vi "pumpsec_09_P2.vi"(0 "reset":i32, 1 "master":i32, 4 "manual":i32, 5 "pause":i32, 10 "Array":dbl[](array[numeric]), 14 "Target":dbl[](array[numeric])=[10.0, 2.0, 0.0, 0.0, 0.0, 0.0, 0.0, 0.0, 0.0, 0.0], 16 "fr_manual":dbl, 17 "Time":dbl[](array[numeric])=[4.0, 2.0, 0.0, 0.0, 0.0, 0.0, 0.0, 0.0, 0.0, 0.0]) -> (2 "pumpCtrl":dbl, 3 "totaltarget":dbl, 6 "target_step":dbl, 7 "REGLO D":dbl, 11 "time_to_target":dbl, 12 "step_fr":dbl, 13 "amount_step":dbl, 19 "reset_out":dbl, 20 "Scale":dbl, 23 "elapsed_step":dbl, 24 "Scale actual":dbl, 25 "params":dbl[](array[numeric]))   [LabVIEW 2016]
uses:
  Desktop/Bertta-Bertta_deploy/Bertta-Bertta_deploy/BERTTA/x64/Debug/BERTTA.dll
panel:
  out "amount_step_previous":dbl
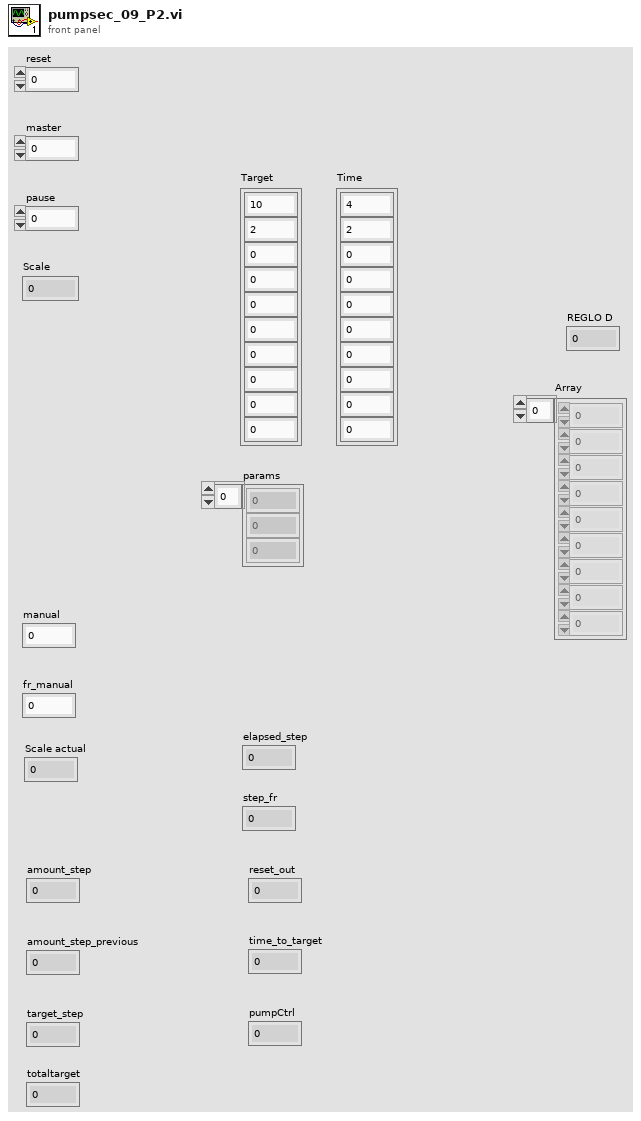
[diagram p1: front panel]
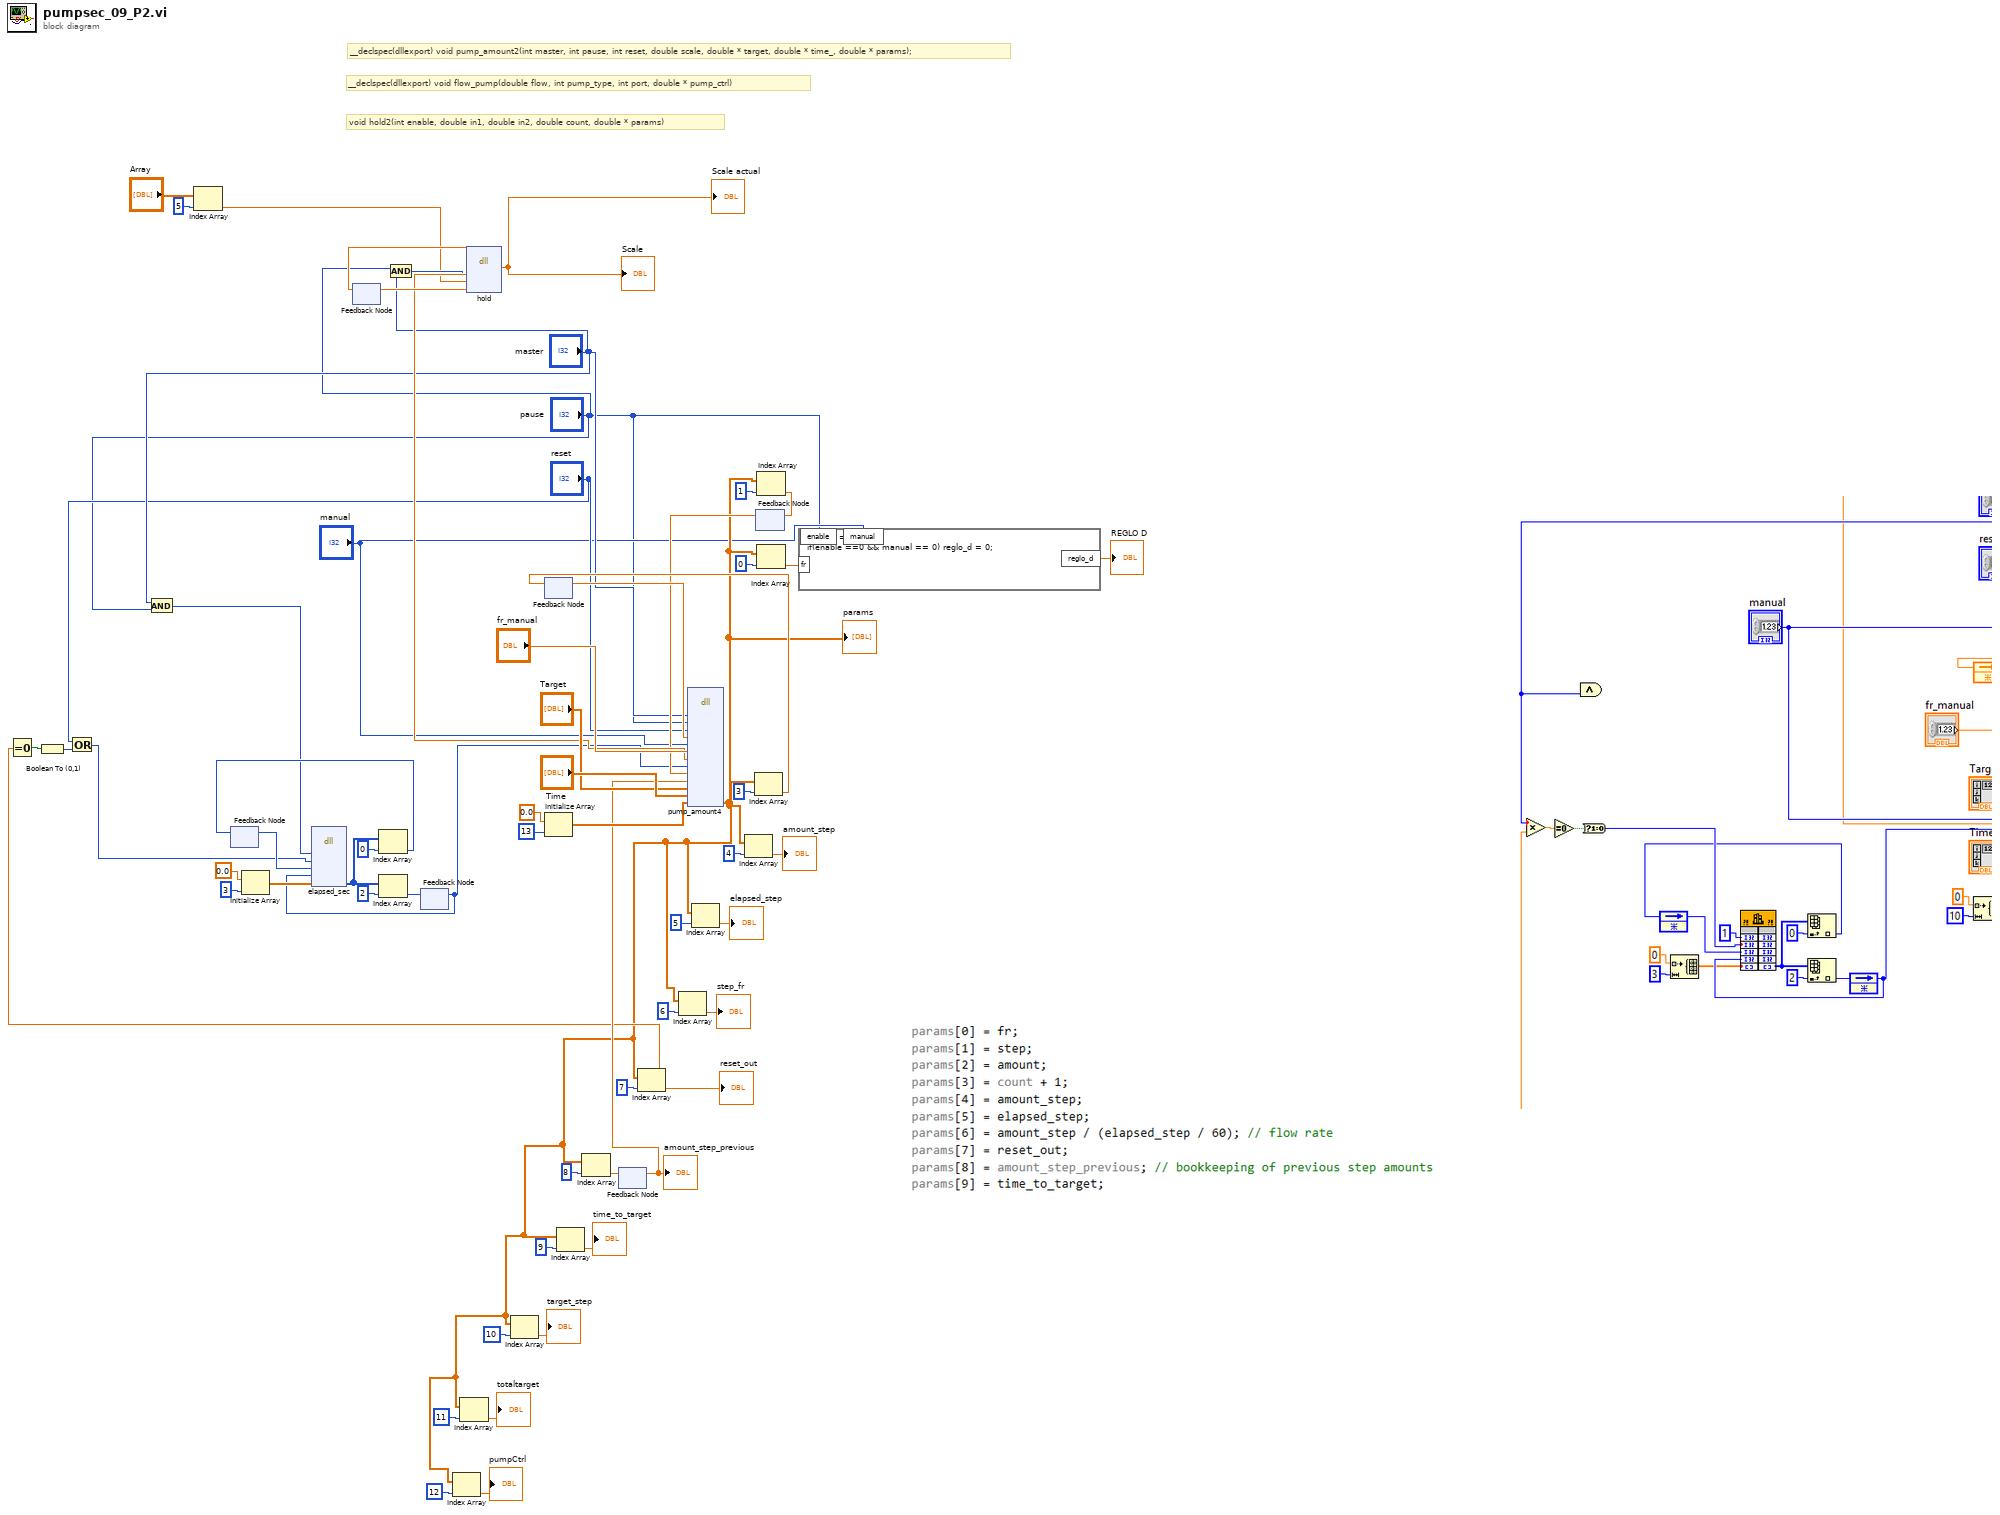
[diagram p0: block diagram]
diagram:
  # "void hold2(int enable, double in1, double in2, double count, double * params)"
  # "__declspec(dllexport) void flow_pump(double flow, int pump_type, int port, double * pump_ctrl)"
  # "__declspec(dllexport) void pump_amount2(int master, int pause, int reset, double scale, double * target, double * time_, double * params);"
  n1 = And(x="master", y="pause") -> (x .and. y?=w20:i32)
  n2 = Index Array(array="Array", index=5) -> (element=w5:dbl)
  n3 = feedback #1() -> (w29:i32)  [unwired: 1 in]
  n4 = Initialize Array(0.0 ("element"), 3 ("dimension size")) -> (w33:dbl[])
  n5 = feedback #2() -> (w52:dbl)  [unwired: 1 in]
  n6 = And(x="pause", y="master") -> (x .and. y?=w50:i32)
  n7 = feedback #3() -> (w27:i32)  [unwired: 1 in]
  n8 = dll-call lib="C:/Users/shresplab/Desktop/Bertta-Bertta_deploy/Bertta-Bertta_deploy/BERTTA/x64/Debug/BERTTA.dll" fn="hold"("enable"=w50, "in1"=w5, "in2"=w52) -> ("return type"=w51:dbl)  [unwired: 6 in, 2 out]
  "Scale" <- w51
  "Scale actual" <- w51
  n9 = feedback-in #2(w51) -> ()
  n10 = feedback #4() -> (w47:dbl)  [unwired: 1 in]
  n11 = Initialize Array(0.0 ("element"), 13 ("dimension size")) -> (w56:dbl[])
  n12 = feedback #5() -> (w24:dbl)  [unwired: 1 in]
  "amount_step_previous" <- w24
  n13 = feedback #6() -> (w37:dbl)  [unwired: 1 in]
  n14 = dll-call lib="C:/Users/shresplab/Desktop/Bertta-Bertta_deploy/Bertta-Bertta_deploy/BERTTA/x64/Debug/BERTTA.dll" fn="pump_amount4"("master"="master", "pause"="pause", "reset"="reset", "count"=w47, "manual"="manual", "fr_manual"="fr_manual", "scale"=w51, "elapsed"=w27, "step_previous"=w37, "amount_step_previous"=w24, "target"="Target", "time_"="Time", "params"=w56) -> ("params"=w8:dbl[])  [unwired: 16 in, 2 out]
  "params" <- w8
  n15 = Index Array(array=w8, index=12) -> (element=→"pumpCtrl":dbl)
  n16 = Index Array(array=w8, index=11) -> (element=→"totaltarget":dbl)
  n17 = Index Array(array=w8, index=10) -> (element=→"target_step":dbl)
  n18 = Index Array(array=w8, index=9) -> (element=→"time_to_target":dbl)
  n19 = Index Array(array=w8, index=8) -> (element=w25:dbl)
  n20 = feedback-in #5(w25) -> ()
  n21 = Index Array(array=w8, index=7) -> (element=w17:dbl)
  "reset_out" <- w17
  n22 = Equal To 0?(x=w17) -> (x = 0?=w16:bool)
  n23 = Boolean To (0,1)(Boolean=w16) -> (0, 1=w15:i16)
  n24 = Or(x="reset", y=w15) -> (x .or. y?=w19:i32)
  n25 = dll-call lib="C:/Users/shresplab/Desktop/Bertta-Bertta_deploy/Bertta-Bertta_deploy/BERTTA/x64/Debug/BERTTA.dll" fn="elapsed_sec"("enable"=w20, "reset"=w19, "last_time"=w29, "elapsed_last"=w27, "params"=w33) -> ("params"=w31:i32[])  [unwired: 8 in, 2 out]
  n26 = Index Array(array=w31, index=0) -> (element=w30:i32)
  n27 = feedback-in #1(w30) -> ()
  n28 = Index Array(array=w31, index=2) -> (element=w28:i32)
  n29 = feedback-in #3(w28) -> ()
  n30 = Index Array(array=w8, index=6) -> (element=→"step_fr":dbl)
  n31 = Index Array(array=w8, index=5) -> (element=→"elapsed_step":dbl)
  n32 = Index Array(array=w8, index=4) -> (element=→"amount_step":dbl)
  n33 = Index Array(array=w8, index=3) -> (element=w48:dbl)
  n34 = feedback-in #4(w48) -> ()
  n35 = Index Array(array=w8, index=1) -> (element=w38:dbl)
  n36 = feedback-in #6(w38) -> ()
  n37 = Index Array(array=w8, index=0) -> (element=w1:dbl)
  n38 = formula code="reglo_d = fr;\nif(enable ==0 && manual == 0) reglo_d = 0;"("enable"="pause", "manual"="manual", "fr"=w1) -> ("reglo_d"=→"REGLO D":dbl)
